vi "Read_Data.vi"(8 "error in (no error)":errorcluster caption="entrée d'erreur (pas d'erreur)", 11 "Firebase PCBA en entrée":refnum<class "Firebase Benches P2193.lvclass">) -> (0 "error out":errorcluster caption="sortie d'erreur", 2 "Data":T1(array[cluster]), 3 "Firebase PCBA en Sortie":refnum<class "Firebase Benches P2193.lvclass">)   [LabVIEW 2020, in "Library Instrument & Equipement.lvlib" / "Library FireBase.lvlib" / "Firebase Benches P2193.lvclass"]
doc: "Returns all data Use Nb_To_Read to determine the number to read\nPlease initialise the following values\n - Name BDD\n - Document\n - API Key\n - Nb To Read"
uses:
  Firebase Benches P2193.lvclass
  Firebase Benches P2193.lvclass/Firebase Benches P2193.ctl
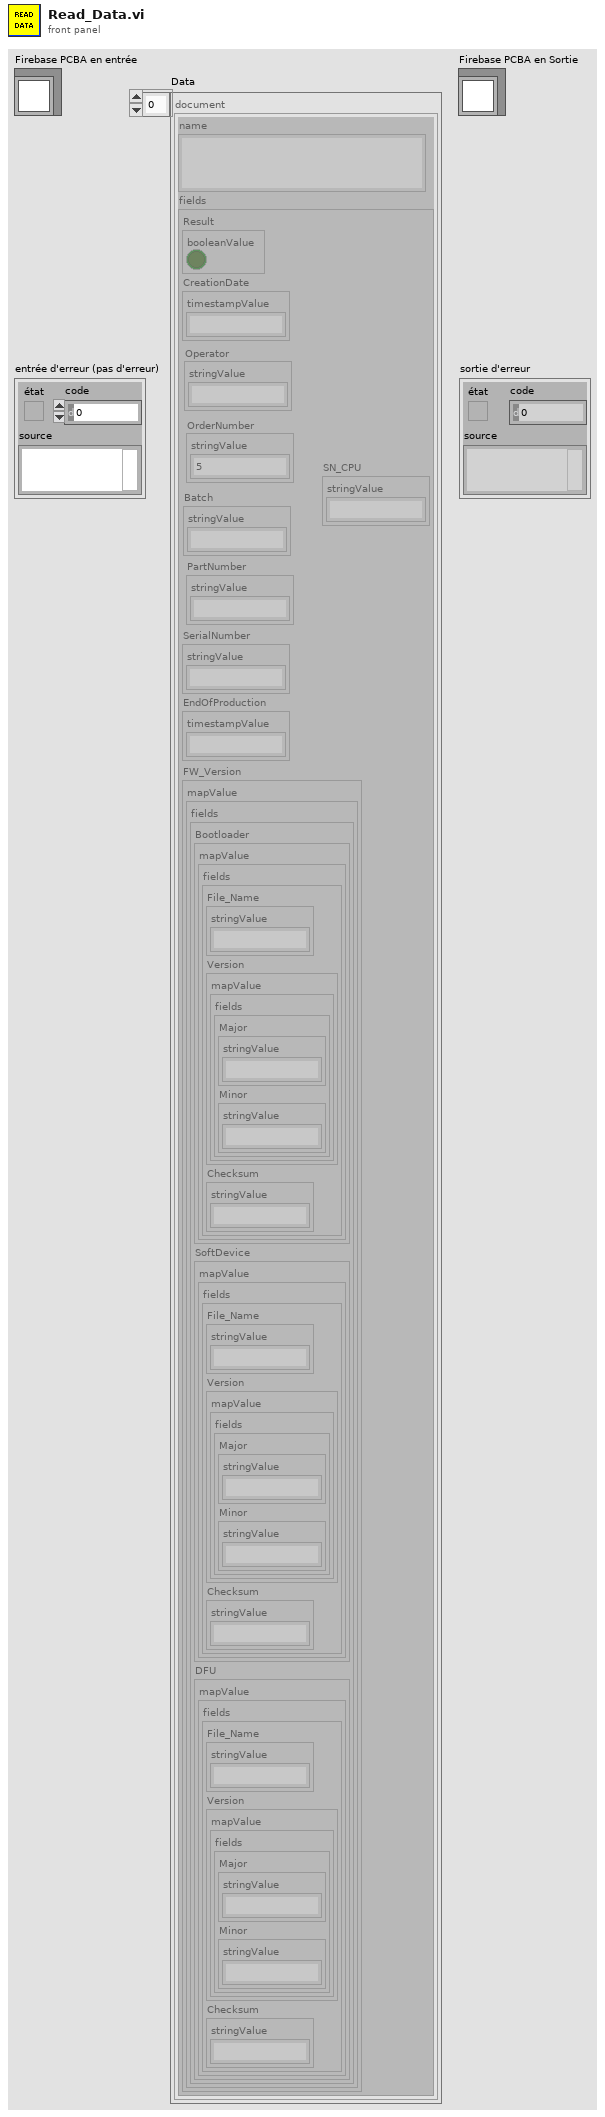
[diagram p1: front panel]
types:
  T1 = cluster{"name":string, "fields":cluster{"Result":cluster{"booleanValue":bool}, "CreationDate":cluster{"timestampValue":string}, "Batch":cluster{"stringValue":string}, "SerialNumber":cluster{"stringValue":string}, "EndOfProduction":cluster{"timestampValue":string}, "FW_Version":cluster{"mapValue":cluster{"fields":cluster{"Bootloader":cluster{"mapValue":cluster{"fields":cluster{"File_Name":cluster{"stringValue":string}, "Version":cluster{"mapValue":cluster{"fields":cluster{"Major":cluster{"stringValue":string}, "Minor":cluster{"stringValue":string}}}}, "Checksum":cluster{"stringValue":string}}}}, "SoftDevice":cluster{"mapValue":cluster{"fields":cluster{"File_Name":cluster{"stringValue":string}, "Version":cluster{"mapValue":cluster{"fields":cluster{"Major":cluster{"stringValue":string}, "Minor":cluster{"stringValue":string}}}}, "Checksum":cluster{"stringValue":string}}}}, "DFU":cluster{"mapValue":cluster{"fields":cluster{"File_Name":cluster{"stringValue":string}, "Version":cluster{"mapValue":cluster{"fields":cluster{"Major":cluster{"stringValue":string}, "Minor":cluster{"stringValue":string}}}}, "Checksum":cluster{"stringValue":string}}}}}}}, "PartNumber":cluster{"stringValue":string}, "OrderNumber":cluster{"stringValue":string}, "Operator":cluster{"stringValue":string}, "SN_CPU":cluster{"stringValue":string}}}[]
  T2 = cluster{"document":cluster{"name":string, "fields":cluster{"Result":cluster{"booleanValue":bool}, "CreationDate":cluster{"timestampValue":string}, "Batch":cluster{"stringValue":string}, "SerialNumber":cluster{"stringValue":string}, "EndOfProduction":cluster{"timestampValue":string}, "FW_Version":cluster{"mapValue":cluster{"fields":cluster{"Bootloader":cluster{"mapValue":cluster{"fields":cluster{"File_Name":cluster{"stringValue":string}, "Version":cluster{"mapValue":cluster{"fields":cluster{"Major":cluster{"stringValue":string}, "Minor":cluster{"stringValue":string}}}}, "Checksum":cluster{"stringValue":string}}}}, "SoftDevice":cluster{"mapValue":cluster{"fields":cluster{"File_Name":cluster{"stringValue":string}, "Version":cluster{"mapValue":cluster{"fields":cluster{"Major":cluster{"stringValue":string}, "Minor":cluster{"stringValue":string}}}}, "Checksum":cluster{"stringValue":string}}}}, "DFU":cluster{"mapValue":cluster{"fields":cluster{"File_Name":cluster{"stringValue":string}, "Version":cluster{"mapValue":cluster{"fields":cluster{"Major":cluster{"stringValue":string}, "Minor":cluster{"stringValue":string}}}}, "Checksum":cluster{"stringValue":string}}}}}}}, "PartNumber":cluster{"stringValue":string}, "OrderNumber":cluster{"stringValue":string}, "Operator":cluster{"stringValue":string}}}}[]
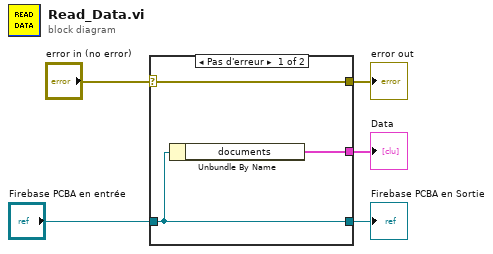
[diagram p0: block diagram]
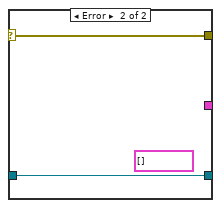
[diagram p2: hidden frame]
diagram:
  n1 = case shown="Pas d'erreur" "error in (no error)" {
    selector: "error in (no error)" -> [w7 w10]
    tunnel: [w7 w10] -> w4
    tunnel: [w6 w9] -> w2
    tunnel: "Firebase PCBA en entrée" -> [w6 w9]
    tunnel: [w8 _] -> w1
    frame No Error {
      n2 = Unbundle By Name(w6) -> ("documents"=w8:T1)
    }
    frame Error {
      (unwired) T2 [] ("Data")
    }
  }
  "error out" <- w4
  "Firebase PCBA en Sortie" <- w2
  "Data" <- w1
